vi "Check Termination Notifiert State.vi"(8 "error in (no error)":errorcluster) -> (0 "error out":errorcluster, 3 "Termination Notifier State":bool)   [LabVIEW 2016]
uses:
  Utilities/Application Globals.vi
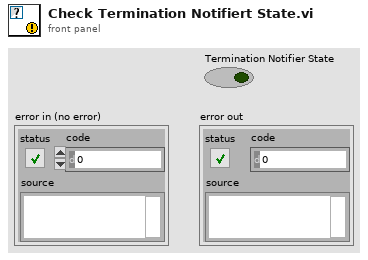
[diagram p1: front panel]
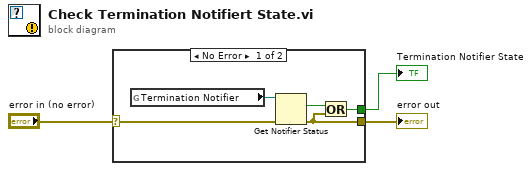
[diagram p0: block diagram]
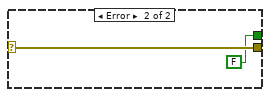
[diagram p2: hidden frame]
diagram:
  n1 = case shown="No Error" "error in (no error)" {
    selector: "error in (no error)" -> [w6 w10]
    tunnel: [w4 w10] -> w3
    tunnel: [w5 FALSE] -> w2
    frame No Error {
      n2 = global read "Application Globals.vi" "Termination Notifier"() -> (w8:refnum<notifier>)
      n3 = Get Notifier Status(notifier=w8, error in (no error)=w6) -> (current notification=w7:bool, error out=w4:errorcluster)  [unwired: 3 out]
      n4 = Or(x=w7, y=w4) -> (x .or. y?=w5:bool)
    }
    frame Error {
    }
  }
  "error out" <- w3
  "Termination Notifier State" <- w2
